vi "XNET IP Stack Wait.vi"(0 "stack in":refnum<k21>, 5 "local interface":string, 7 "timeout ms (60000)":i32=60000, 11 "error in":errorcluster) -> (4 "stack out":refnum<k21>, 15 "error out":errorcluster)   [LabVIEW 2018]
doc: "Waits for interface(s) in the XNET IP Stack to be ready for communication."
uses:
  nixlvapi.dll
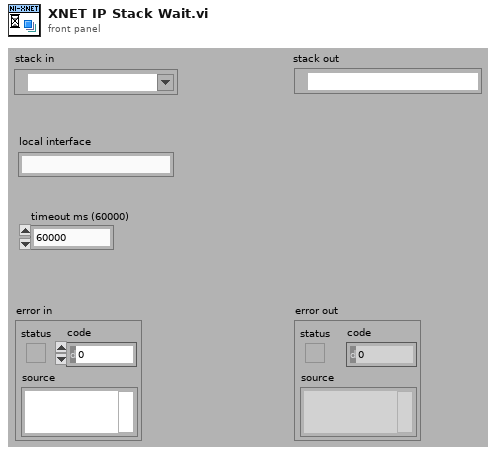
[diagram p1: front panel]
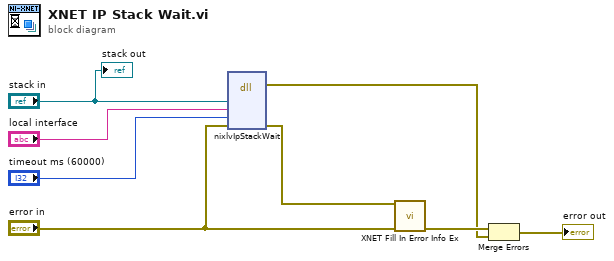
[diagram p0: block diagram]
diagram:
  n1 = dll-call lib="nixlvapi.*" fn="nixlvIpStackWait" label="Call Library"("reference"="stack in", "localInterface"="local interface", "timeoutMs"="timeout ms (60000)", "errorInOut"="error in") -> (error out=w6:errorcluster, "errorInOut"=w8:errorcluster)  [unwired: 3 in, 5 out]
  n2 = call "XNET Fill In Error Info Ex.vi"("error xnet"=w8, "error in"="error in") -> ("error out"=w7:errorcluster)  [unwired: 13 in]
  n3 = Merge Errors(w7, w6) -> (→"error out":errorcluster)
  "stack out" <- "stack in"
